vi "SweepCtrlDeltaCurrent_ver2.0.vi"(5 "# of pts discarded":i32=3, 7 "Keithley 6221":T1={"Delta "=FALSE, "Const I "=FALSE, "Pulse Delta "=FALSE, "Sine Wave "=FALSE, "From I_HI (A)"=0.0, "From I (A)"=0.0, "I_LO (A)"=0.0, "From I_H (A)"=0.0, "I_L (A)"=0.0, "Freq (Hz)"=13.259, "From I_Sin (A)"=0.0, "DC Offset (A)"=0.0, "Delay Time (s)"=1.0, "Pulse Width (s)"=0.012, "Delay (s)"=0.011966, "To I (A)"=0.0, "ASymmetric?"=FALSE, "To I_HI (A)"=0.0, "To I_H (A)"=0.0, "To I_Sin (A)"=0.0, "GPIB ADR"=0, "Sweep Mode"=0, "Delta Unit"="V", "2182A range (V)"=0.01, "6221 Compliance (V)"=10.0} {"Sweep Mode" items=["Linear", "Log", "Exp", "Inverse", "Manual"]; "GPIB ADR" items=["None"=0, "12"=12, "13"=13]; "To I_Sin (A)" format="%#.5p"; "To I_H (A)" format="%#.5p"; "To I_HI (A)" format="%#.5p"; "To I (A)" format="%#.5p"; "Delay (s)" format="%.3p"; "Pulse Width (s)" format="%.3p"; "Delay Time (s)" format="%#.5p"; "DC Offset (A)" format="%#.5p"; "From I_Sin (A)" format="%#.5p"; "Freq (Hz)" format="%#_6p"; "I_L (A)" format="%#.5p"; "From I_H (A)" format="%#.5p"; "I_LO (A)" format="%#.5p"; "From I (A)" format="%#.5p"; "From I_HI (A)" format="%#.5p"}, 8 "error in (no error)":errorcluster, 9 "Set pt change flag":bool, 10 "DC St. Pt.":dbl, 11 "GPIB ADR":u16) -> (0 "error out":errorcluster)   [LabVIEW 2012]
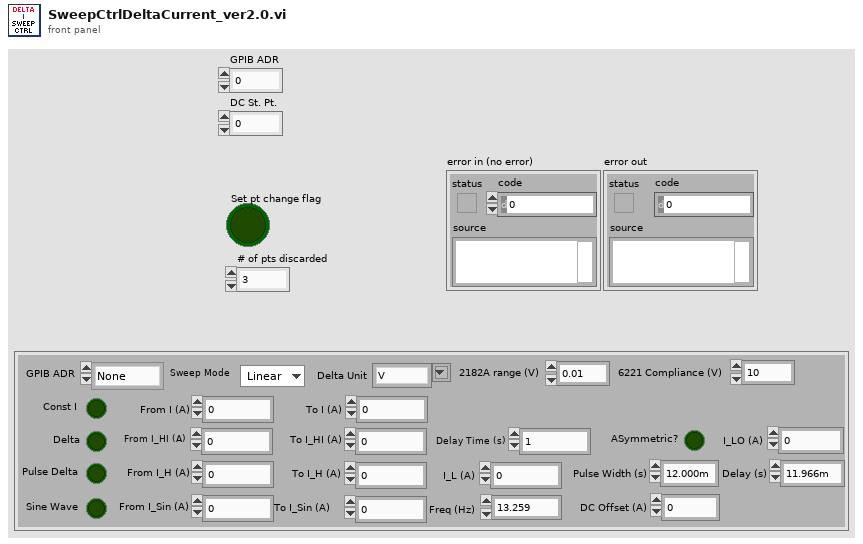
[diagram p1: front panel]
types:
  T1 = cluster{"Delta ":bool, "Const I ":bool, "Pulse Delta ":bool, "Sine Wave ":bool, "From I_HI (A)":dbl, "From I (A)":dbl, "I_LO (A)":dbl, "From I_H (A)":dbl, "I_L (A)":dbl, "Freq (Hz)":dbl, "From I_Sin (A)":dbl, "DC Offset (A)":dbl, "Delay Time (s)":dbl, "Pulse Width (s)":dbl, "Delay (s)":dbl, "To I (A)":dbl, "ASymmetric?":bool, "To I_HI (A)":dbl, "To I_H (A)":dbl, "To I_Sin (A)":dbl, "GPIB ADR":u16, "Sweep Mode":u8, "Delta Unit":string, "2182A range (V)":dbl, "6221 Compliance (V)":dbl}
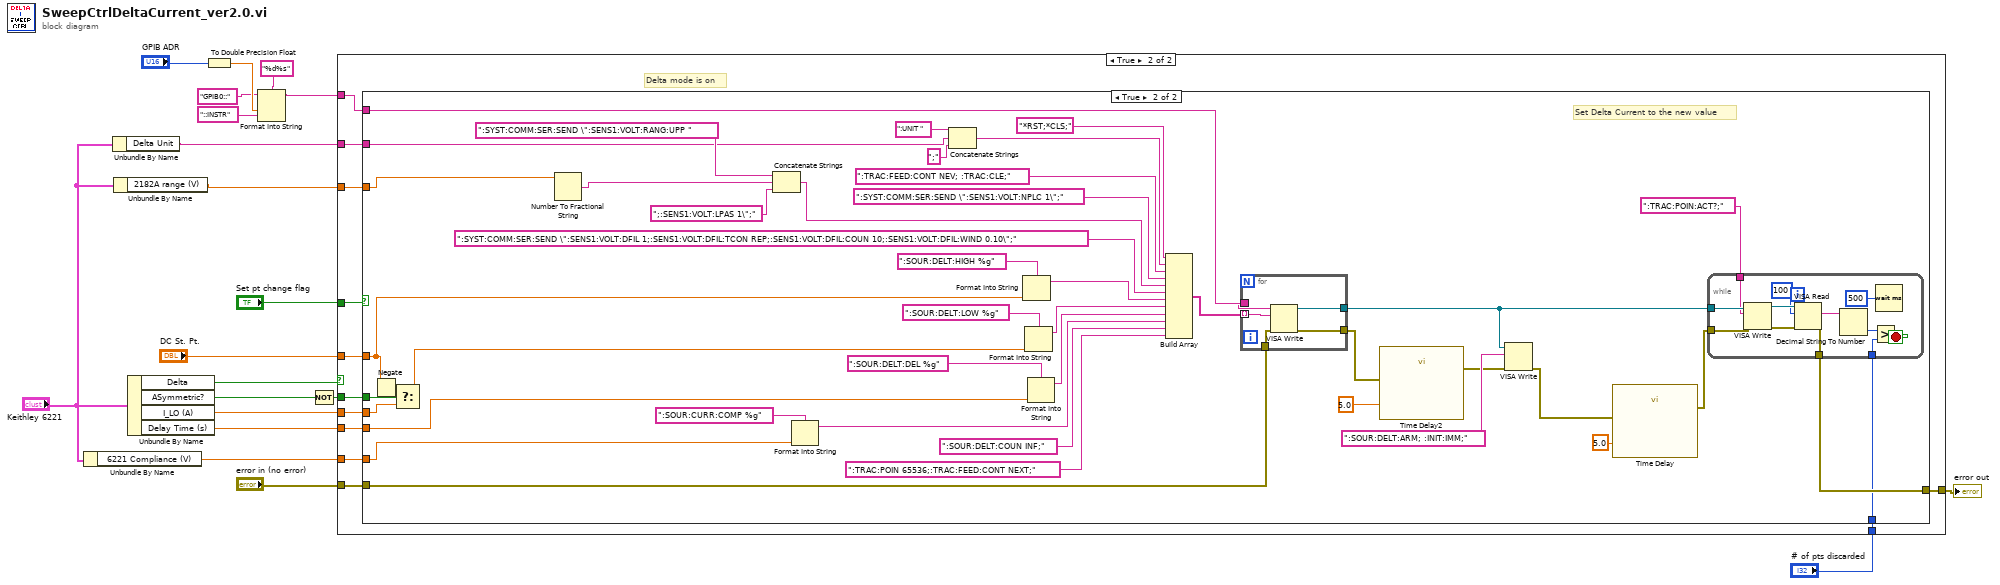
[diagram p0: block diagram]
diagram:
  n1 = Unbundle By Name("Keithley 6221") -> ("6221 Compliance (V)"=w3:dbl)
  n2 = Unbundle By Name("Keithley 6221") -> ("Delta Unit"=w1:string)
  n3 = Unbundle By Name("Keithley 6221") -> ("2182A range (V)"=w4:dbl)
  n4 = Unbundle By Name("Keithley 6221") -> ("Delta"=w15:bool, "ASymmetric?"=w12:bool, "I_LO (A)"=w11:dbl, "Delay Time (s)"=w9:dbl)
  n5 = To Double Precision Float(number="GPIB ADR") -> (double precision float=w19:dbl)
  n6 = Format Into String(format string="%d%s" ("Removes all labels from the string"), initial string="GPIB0::", w19, "::INSTR") -> (resulting string=w14:string)  [unwired: 1 in, 1 out]
  n7 = Not(x=w12) -> (.not. x?=w10:bool)
  n8 = case shown="True" w15 {
    tunnel: "Set pt change flag" -> [_ w33]
    tunnel: w14 -> [_ w32]
    tunnel: "DC St. Pt." -> [_ w31]
    tunnel: w10 -> [_ w30]
    tunnel: w11 -> [_ w29]
    tunnel: w9 -> [_ w28]
    tunnel: "error in (no error)" -> [w21 w27]
    tunnel: [w21 w26] -> w7
    tunnel: "# of pts discarded" -> [_ w25]
    tunnel: w4 -> [_ w24]
    tunnel: w3 -> [_ w23]
    tunnel: w1 -> [_ w22]
    frame False {
      # "Delta mode is off"
    }
    frame True {
      # "Delta mode is on"
      n9 = case shown="True" w33 {
        tunnel: w32 -> [_ w76]
        tunnel: w31 -> [_ w66]
        tunnel: w30 -> [_ w67]
        tunnel: w29 -> [_ w65]
        tunnel: w28 -> [_ w62]
        tunnel: w27 -> [w34 w56]
        tunnel: [w34 w54] -> w26
        tunnel: w25 -> [_ w53]
        tunnel: w24 -> [_ w39]
        tunnel: w23 -> [_ w36]
        tunnel: w22 -> [_ w35]
        frame False {
          # "Set Values are not changed"
        }
        frame True {
          # "Set Delta Current to the new value"
          n10 = Negate(x=w66) -> (-x=w52:dbl)
          n11 = Select(t=w52, s=w67, f=w65) -> (s? t:f=w64:dbl)
          n12 = Number To Fractional String(number=w39) -> (F-format string=w42:string)  [unwired: 3 in]
          n13 = Concatenate Strings(":SYST:COMM:SER:SEND \":SENS1:VOLT:RANG:UPP " ("format string"), w42, ";:SENS1:VOLT:LPAS 1\";" ("format string")) -> (w40:string)
          n14 = Format Into String(format string=":SOUR:CURR:COMP %g", w36) -> (resulting string=w37:string)  [unwired: 2 in, 1 out]
          n15 = Concatenate Strings(":UNIT " ("write buffer"), w35, ";" ("string")) -> (w74:string)
          n16 = Format Into String(format string=":SOUR:DELT:HIGH %g", w66) -> (resulting string=w69:string)  [unwired: 2 in, 1 out]
          n17 = Format Into String(format string=":SOUR:DELT:LOW %g", w64) -> (resulting string=w61:string)  [unwired: 2 in, 1 out]
          n18 = Format Into String(format string=":SOUR:DELT:DEL %g", w62) -> (resulting string=w60:string)  [unwired: 2 in, 1 out]
          n19 = Build Array("*RST;*CLS;" ("write buffer"), w74, ":TRAC:FEED:CONT NEV; :TRAC:CLE;" ("format string"), ":SYST:COMM:SER:SEND \":SENS1:VOLT:NPLC 1\";", w40, ":SYST:COMM:SER:SEND \":SENS1:VOLT:DFIL 1;:SENS1:VOLT:DFIL:TCON REP;:SENS1:VOLT:DFIL:COUN 10;:SENS1:VOLT:DFIL:WIND 0.10\";", w69, w61, w60, w37, ":SOUR:DELT:COUN INF;", ":TRAC:POIN 65536;:TRAC:FEED:CONT NEXT;" ("format string")) -> (w57:string[])
          n20 = for {
            tunnel: w57 -> [w95] mode=indexing
            tunnel: w76 -> [w94]
            tunnel: [w93] -> w45
            tunnel: w56 -> [w92]
            tunnel: [w91] -> w49
            n21 = VISA Write(VISA resource name=w94, write buffer=w95, error in (no error)=w92) -> (VISA resource name out=w91:refnum<visa-resource-name>, error out=w93:errorcluster)  [unwired: 1 out]
          }
          n22 = call "Time Delay2"("error in (no error)"=w45, "Delay Time (s)"=5.0) -> ("error out"=w46:errorcluster)  [unwired: 9 in]
          n23 = VISA Write(VISA resource name=w49, write buffer=":SOUR:DELT:ARM; :INIT:IMM;" ("format string"), error in (no error)=w46) -> (error out=w47:errorcluster)  [unwired: 2 out]
          n24 = call "Time Delay"("error in (no error)"=w47, "Delay Time (s)"=5.0) -> ("error out"=w51:errorcluster)  [unwired: 9 in]
          n25 = while {
            tunnel: w49 -> [w90]
            tunnel: w51 -> [w89]
            tunnel: ":TRAC:POIN:ACT?;" ("write buffer") -> [w88]
            tunnel: [w81] -> w54
            tunnel: w53 -> [w79]
            stop <- w82 stop-if-true
            n26 = VISA Write(VISA resource name=w90, write buffer=w88, error in (no error)=w89) -> (VISA resource name out=w86:refnum<visa-resource-name>, error out=w87:errorcluster)  [unwired: 1 out]
            n27 = VISA Read(VISA resource name=w86, byte count=u32 100, error in (no error)=w87) -> (read buffer=w84:string, error out=w81:errorcluster)  [unwired: 2 out]
            n28 = Decimal String To Number(string=w84) -> (number=w83:i32)  [unwired: 2 in, 1 out]
            n29 = Greater?(x=w83, y=w79) -> (0:w82:bool)
            n30 = Wait (ms)(milliseconds to wait=u32 500) -> ()  [unwired: 1 out]
          }
        }
      }
    }
  }
  "error out" <- w7
